vi "Lookup.vi"(7 "Action":T1, 8 "error in (no error)":errorcluster, 10 "Top Level VI":string) -> (0 "error out":errorcluster, 2 "Counter":refnum<class "Panel Control Counter.lvclass">)   [LabVIEW 2020, in "Panel.lvlib" / "Cursor.lvclass"]
doc: "Looks up the current Control Counter\n\n----\nPlease see the following web address for additional documentation and tutorial information:\nhttp://www.mooregoodideas.com/mgi-panel-manager/\n\nAuthor: Derek Trepanier\n\nCopyright (c) 2018, Moore Good Ideas, Inc.\n\nAll rights reserved.\n\nRedistribution and use in source and binary forms, with or without modification, are permitted provided that the following conditions are met:\n\n * Redistributions of source code must retain the above copyright notice, this list of conditions and the following disclaimer.\n * Redistributions in binary form must reproduce the above copyright notice, this list of conditions and the following disclaimer in the documentation and/or other materials provided with the distribution.\n * Neither the name of Moore Good Ideas, Inc. nor the names of its contributors may be used to endorse or promote products derived from this software without specific prior written permission.\n\nTHIS SOFTWARE IS PROVIDED BY THE COPYRIGHT HOLDERS AND CONTRIBUTORS \"AS IS\" AND ANY EXPRESS OR IMPLIED WARRANTIES, INCLUDING, BUT NOT LIMITED TO, THE IMPLIED WARRANTIES OF MERCHANTABILITY AND FITNESS FOR A PARTICULAR PURPOSE ARE DISCLAIMED. IN NO EVENT SHALL THE COPYRIGHT OWNER OR CONTRIBUTORS BE LIABLE FOR ANY DIRECT, INDIRECT, INCIDENTAL, SPECIAL, EXEMPLARY, OR CONSEQUENTIAL DAMAGES (INCLUDING, BUT NOT LIMITED TO, PROCUREMENT OF SUBSTITUTE GOODS OR SERVICES; LOSS OF USE, DATA, OR PROFITS; OR BUSINESS INTERRUPTION) HOWEVER CAUSED AND ON ANY THEORY OF LIABILITY, WHETHER IN CONTRACT, STRICT LIABILITY, OR TORT (INCLUDING NEGLIGENCE OR OTHERWISE) ARISING IN ANY WAY OUT OF THE USE OF THIS SOFTWARE, EVEN IF ADVISED OF THE POSSIBILITY OF SUCH DAMAGE."
uses:
  <vilib>/MGI/Panel Manager/Panel/Cursor/Cursor.lvclass
  <vilib>/MGI/Panel Manager/Panel/Cursor/Lookup Actions.ctl
  <vilib>/MGI/Panel Manager/Panel/Panel Control Counter/Panel Control Counter.lvclass
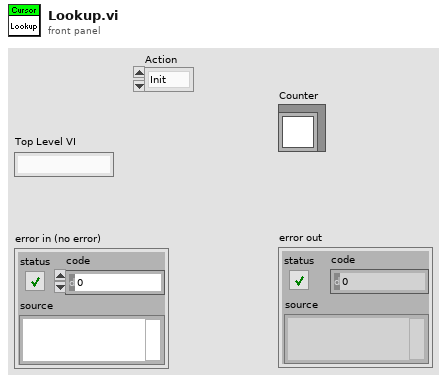
[diagram p1: front panel]
types:
  T1 = typedef "Panel.lvlib/Cursor.lvclass/Lookup Actions.ctl" = enum16{"Init", "Get", "Destroy"}
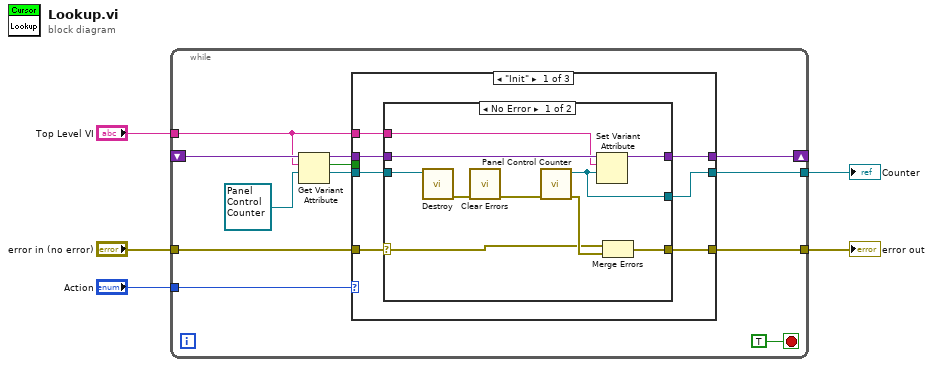
[diagram p0: block diagram]
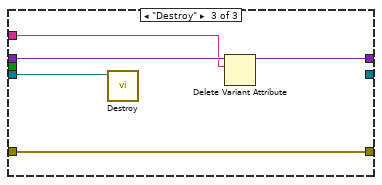
[diagram p4: hidden frame]
diagram:
  n1 = while {
    shift-right: [w15] -> _
    shift-left: _ -> [w17]
    tunnel: "Action" -> [w11]
    tunnel: [w10] -> w4
    tunnel: "Top Level VI" -> [w8]
    tunnel: "error in (no error)" -> [w7]
    tunnel: [w6] -> w1
    stop <- TRUE stop-if-true
    n2 = Get Variant Attribute(Variant=w17, name=w8, default value (empty Variant)=refnum<class "Panel Control Counter.lvclass"> refnum ("Panel.lvlib:Panel Control Counter.lvclass")) -> (duplicate Variant=w14:variant, found=w13:bool, value=w12:refnum<class "Panel Control Counter.lvclass">)  [unwired: 1 in, 1 out]
    n3 = case shown="\"Init\"" w11 {
      tunnel: [w22 w39 w41] -> w15
      tunnel: w14 -> [w24 w39 w44]
      tunnel: w12 -> [w23 w38 w42]
      tunnel: w13 -> [_ _ _]
      tunnel: [w20 w38 _] -> w10
      tunnel: w8 -> [w21 _ w40]
      tunnel: w7 -> [w19 w37 w43]
      tunnel: [w18 w37 w43] -> w6
      frame "Init" {
        n4 = case shown="No Error" w19 {
          selector: w19 -> [w25 w35]
          tunnel: w24 -> [w34 w36]
          tunnel: w23 -> [w33 _]
          tunnel: [w32 w36] -> w22
          tunnel: w21 -> [w31 _]
          tunnel: [w28 _] -> w20
          tunnel: [w26 w35] -> w18
          frame No Error {
            n5 = call <vilib>:"Destroy.vi"("Panel Control Counter in"=w33) -> ("error out"=w30:errorcluster)  [unwired: 10 in]
            n6 = call <vilib>:"Clear Errors.vi"("error in (no error)"=w30) -> ("error out"=w29:errorcluster)  [unwired: 5 in, 1 out]
            n7 = call <vilib>:"Panel Control Counter.vi"("error in (no error)"=w29) -> ("error out"=w27:errorcluster, "Panel Control Counter out"=w28:refnum<class "Panel Control Counter.lvclass">)  [unwired: 9 in]
            n8 = Set Variant Attribute(Variant=w34, name=w31, value=w28) -> (Variant out=w32:variant)  [unwired: 1 in, 2 out]
            n9 = Merge Errors(w25, w27) -> (w26:errorcluster)
          }
          frame Error {
          }
        }
      }
      frame "Get" {
      }
      frame "Destroy" {
        n10 = call <vilib>:"Destroy.vi"("Panel Control Counter in"=w42) -> ()  [unwired: 10 in, 1 out]
        n11 = Delete Variant Attribute(6:w40, 7:w44) -> (3:w41:variant)  [unwired: 1 in, 2 out]
      }
    }
  }
  "Counter" <- w4
  "error out" <- w1
